vi "VelocityAndFreq_APT.vi"(5 "Points per burst":i32=200, 6 "Picture in":refnum<vi>, 7 "Max frequency [Hz]":dbl=200.0, 10 "CurrenMeters":cluster{"Array":timestamp[], "Array":dbl[]}[](array[cluster]), 11 "Specs_time":cluster{"Waveform":waveform(dbl), timestamp}[](array[cluster])) -> ()   [LabVIEW 2016]
uses:
  <vilib>/Heliosphere Research LLC/Advanced Plotting Toolkit/Advanced Plotting Toolkit.lvlib
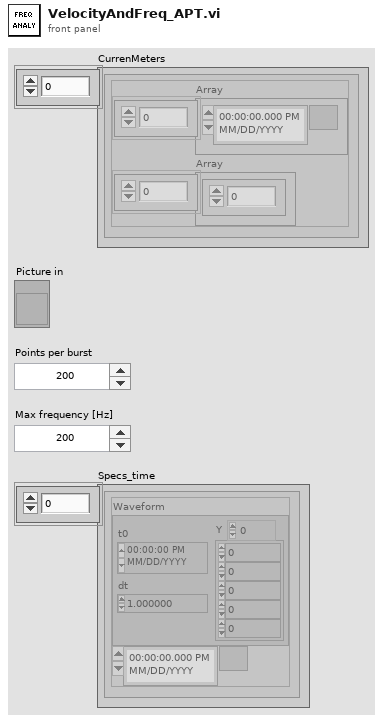
[diagram p1: front panel]
types:
  T1 = typedef "Advanced Plotting Toolkit.lvlib/PlotID.ctl" = i32
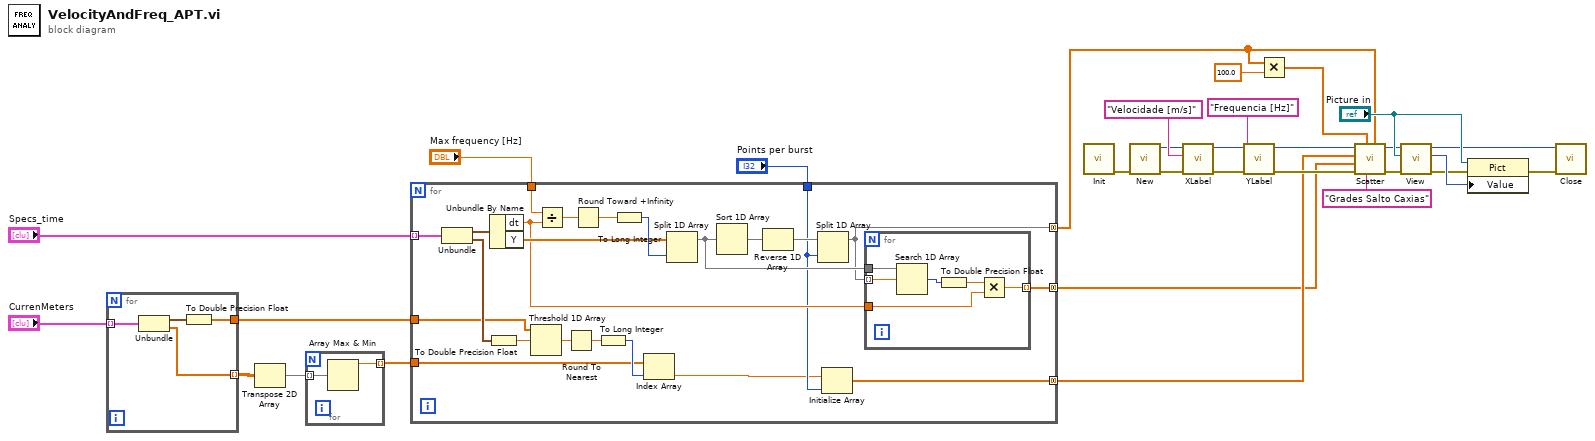
[diagram p0: block diagram]
diagram:
  n1 = for {
    tunnel: "CurrenMeters" -> [w34] mode=indexing
    tunnel: [w32] -> w11
    tunnel: [w31] -> w8 mode=indexing
    n2 = Unbundle(w34) -> ("Array"=w33:timestamp[], "Array"=w31:dbl[])
    n3 = To Double Precision Float(number=w33) -> (double precision float=w32:dbl[])
  }
  n4 = Transpose 2D Array(2D array=w8) -> (transposed array=w9:dbl[][])
  n5 = for {
    tunnel: w9 -> [w36] mode=indexing
    tunnel: [w35] -> w12 mode=indexing
    n6 = Array Max & Min(array=w36) -> (max value=w35:dbl)  [unwired: 3 out]
  }
  n7 = for {
    tunnel: "Specs_time" -> [w59] mode=indexing
    tunnel: "Max frequency [Hz]" -> [w57]
    tunnel: [w40] -> w24 mode=concatenating
    tunnel: [w51] -> w3 mode=concatenating
    tunnel: w11 -> [w46]
    tunnel: w12 -> [w44]
    tunnel: [w37] -> w4 mode=concatenating
    tunnel: "Points per burst" -> [w39]
    n8 = Unbundle(w59) -> ("Waveform"=w58:waveform(dbl), w47:timestamp)
    n9 = To Double Precision Float(number=w47) -> (double precision float=w48:dbl)
    n10 = Unbundle By Name(w58) -> ("dt"=w52:dbl, "Y"=w53:dbl[])
    n11 = Threshold 1D Array(2:w48, 3:w46) -> (0:w49:dbl)  [unwired: 1 in]
    n12 = Divide(x=w57, y=w52) -> (x/y=w56:dbl)
    n13 = Round To Nearest(number=w49) -> (nearest integer value=w50:dbl)
    n14 = Round Toward +Infinity(x=w56) -> (ceil(x): smallest int >= x=w55:dbl)
    n15 = To Long Integer(number=w50) -> (32bit integer=w45:i32)
    n16 = To Long Integer(number=w55) -> (32bit integer=w54:i32)
    n17 = Index Array(array=w44, index=w45) -> (element=w38:dbl)
    n18 = Split 1D Array(array=w53, index=w54) -> (first subarray=w41:dbl[])  [unwired: 1 out]
    n19 = Sort 1D Array(array=w41) -> (sorted array=w43:dbl[])
    n20 = Reverse 1D Array(array=w43) -> (reversed array=w42:dbl[])
    n21 = Split 1D Array(array=w42, index=w39) -> (first subarray=w40:dbl[])  [unwired: 1 out]
    n22 = Initialize Array(w38, w39) -> (w37:dbl[])
    n23 = for {
      tunnel: w52 -> [w64]
      tunnel: [w63] -> w51 mode=indexing
      tunnel: w41 -> [w62]
      tunnel: w40 -> [w61] mode=indexing
      n24 = Search 1D Array(1D array=w62, element=w61) -> (index of element=w60:i32)  [unwired: 1 in]
      n25 = To Double Precision Float(number=w60) -> (double precision float=w65:dbl)
      n26 = Multiply(x=w65, y=w64) -> (x*y=w63:dbl)
    }
  }
  n27 = call <vilib>:"Init.vi"() -> ("error out"=w5:errorcluster)  [unwired: 11 in]
  n28 = call <vilib>:"New.vi"("error in (no error)"=w5) -> ("error out"=w18:errorcluster, "Plot ID"=w19:T1)  [unwired: 9 in]
  n29 = call <vilib>:"XLabel.vi"("error in (no error)"=w18, "Label"="Velocidade [m/s]", "Plot ID"=w19) -> ("error out"=w17:errorcluster, "Plot ID out"=w16:T1)  [unwired: 7 in]
  n30 = call <vilib>:"YLabel.vi"("error in (no error)"=w17, "Label"="Frequencia [Hz]", "Plot ID"=w16) -> ("error out"=w21:errorcluster, "Plot ID out"=w20:T1)  [unwired: 7 in]
  n31 = Multiply(x=w24, y=100.0) -> (x*y=w26:dbl[])
  n32 = call <vilib>:"Scatter.vi"("Colormap Values"=w24, "Legend Title"="Grades Salto Caxias", "Areas"=w26, "error in (no error)"=w21, "Y Data"=w3, "X Data"=w4, "Plot ID"=w20) -> ("error out"=w13:errorcluster, "Plot ID Out"=w14:T1)  [unwired: 3 in]
  n33 = call <vilib>:"View.vi"("error in (no error)"=w13, "Ref for Sizing"="Picture in", "Plot ID"=w14) -> ("error out"=w28:errorcluster, "Picture"=w30:picture, "Plot ID Out"=w1:T1)  [unwired: 6 in]
  n34 = property class="Pict"(reference="Picture in", error in=w28, "Value"=w30) -> (error out=w2:errorcluster)  [unwired: 1 out]
  n35 = call <vilib>:"Close.vi"("error in (no error)"=w2, "Plot ID"=w1) -> ()  [unwired: 9 in, 1 out]
